vi "Resolve Link.vi"   [LabVIEW 2018, in "Toolkit.lvlib" / "SFTP.lvclass"]
uses:
  SFTP.lvclass
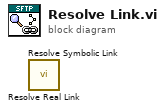
[diagram p0: block diagram]
diagram:
  n1 = call "Resolve Real Link.vi"() -> ()  [unwired: 9 in, 3 out]
  n2 = call "Resolve Symbolic Link.vi"() -> ()  [unwired: 9 in, 3 out]
